vi "S2C_VLFT10_Proc_BoardPresent.vi"(8 "Error In":errorcluster, 11 "HandSwitch":T1 items=["Mono1 Cut", "Mono1 Coag", "Mono2 Cut", "Mono2 Coag", "Mono2 ValleyLab", "Bipolar", "LXF Bipolar", "Ligasure", "LXF Ligasure"]) -> (0 "Error Out":errorcluster, 3 "Present?":bool)   [LabVIEW 2015]
uses:
  Typedefs/S2C_VLFT10_Type_HandSwitch.ctl
  PCIe7841/VIs/Typedefs/S2C_PCIe7841_Type_PathRelayRd.ctl
  PCIe7841/VIs/Typedefs/S2C_PCIe7841_Type_RemRd.ctl
  PCIe7841/VIs/Typedefs/S2C_PCIe7841_Type_HandSwitchRd.ctl
  PCIe7841/VIs/Typedefs/S2C_PCIe7841_Type_SmokeEvacRd.ctl
  PCIe7841/VIs/PolyDriver/S2C_PCIe7841_Poly_RelayPathRead.vi
  PCIe7841/VIs/PolyDriver/S2C_PCIe7841_Poly_RemRead.vi
  PCIe7841/VIs/PolyDriver/S2C_PCIe7841_Poly_HandSwitchRead.vi
  PCIe7841/VIs/PolyDriver/S2C_PCIe7841_Poly_SmokeEvacRead.vi
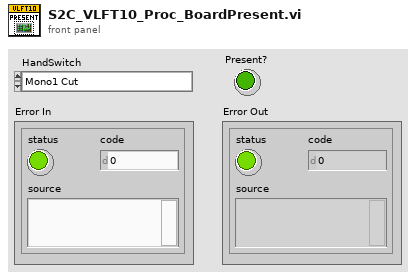
[diagram p1: front panel]
types:
  T1 = typedef "S2C_VLFT10_Type_HandSwitch.ctl" = u16
  T2 = typedef "S2C_PCIe7841_Type_HandSwitchRd.ctl" = string
  T3 = typedef "S2C_PCIe7841_Type_RemRd.ctl" = string
  T4 = typedef "S2C_PCIe7841_Type_PathRelayRd.ctl" = string
  T5 = typedef "S2C_PCIe7841_Type_SmokeEvacRd.ctl" = string
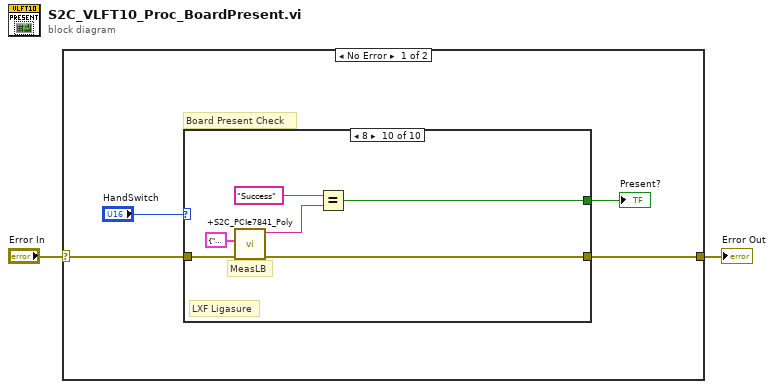
[diagram p0: block diagram]
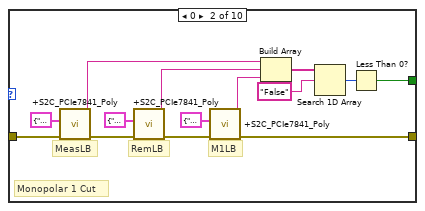
[diagram p3: hidden frame]
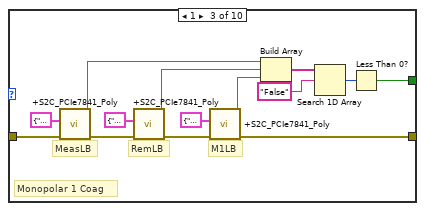
[diagram p4: hidden frame]
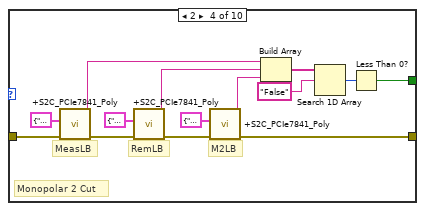
[diagram p5: hidden frame]
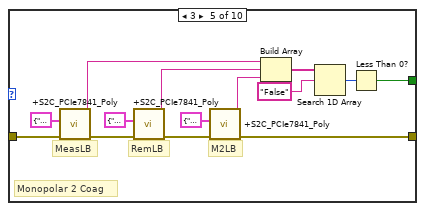
[diagram p6: hidden frame]
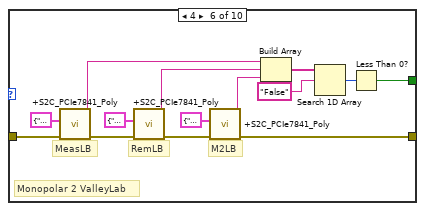
[diagram p7: hidden frame]
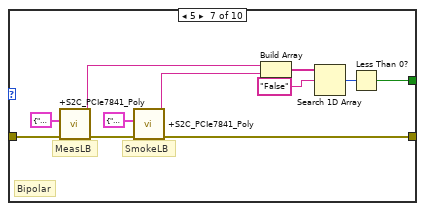
[diagram p8: hidden frame]
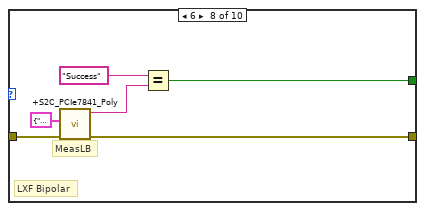
[diagram p9: hidden frame]
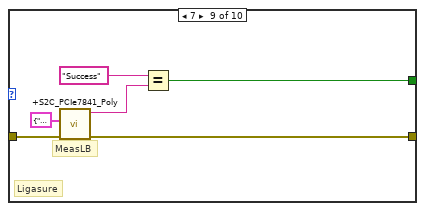
[diagram p10: hidden frame]
diagram:
  n1 = case shown="No Error" "Error In" {
    selector: "Error In" -> [w5 w107]
    tunnel: [w3 w107] -> w2
    frame No Error {
      # "Board Present Check"
      n2 = case shown="8" "HandSwitch" {
        tunnel: w5 -> [w7 w18 w32 w46 w60 w74 w87 w93 w99 w105]
        tunnel: [w7 w9 w23 w37 w51 w65 w79 w89 w95 w101] -> w3
        tunnel: [_ w8 w22 w36 w50 w64 w80 w92 w98 w104] -> w4
        frame 99, Default {
        }
        frame 0 {
          # "Monopolar 1 Cut"
          # "M1LB"
          # "RemLB"
          # "MeasLB"
          n3 = call-poly "+S2C_PCIe7841_Poly.vi"("Error In"=w18, "RelayPath"=cluster{"RelayPath":T4} {"RelayPath"="143"}) -> ("Error Out"=w17:errorcluster, "Response"=w15:string)  [unwired: 8 in]
          n4 = call-poly "+S2C_PCIe7841_Poly.vi"("Error In"=w17, "REM"=cluster{"REM":T3} {"REM"="123"}) -> ("Error Out"=w16:errorcluster, "Response"=w14:string)  [unwired: 8 in]
          n5 = call-poly "+S2C_PCIe7841_Poly.vi"("Error In"=w16, "HandSwitch"=cluster{"HandSwitch":T2} {"HandSwitch"="127"}) -> ("Error Out"=w9:errorcluster, "Response"=w13:string)  [unwired: 8 in]
          n6 = Build Array(w15, w14, w13) -> (w12:string[])
          n7 = Search 1D Array(1D array=w12, element="False") -> (index of element=w10:i32)  [unwired: 1 in]
          n8 = Less Than 0?(x=w10) -> (x < 0?=w8:bool)
        }
        frame 1 {
          # "Monopolar 1 Coag"
          # "M1LB"
          # "RemLB"
          # "MeasLB"
          n9 = call-poly "+S2C_PCIe7841_Poly.vi"("Error In"=w32, "RelayPath"=cluster{"RelayPath":T4} {"RelayPath"="143"}) -> ("Error Out"=w31:errorcluster, "Response"=w29:string)  [unwired: 8 in]
          n10 = call-poly "+S2C_PCIe7841_Poly.vi"("Error In"=w31, "REM"=cluster{"REM":T3} {"REM"="123"}) -> ("Error Out"=w30:errorcluster, "Response"=w28:string)  [unwired: 8 in]
          n11 = call-poly "+S2C_PCIe7841_Poly.vi"("Error In"=w30, "HandSwitch"=cluster{"HandSwitch":T2} {"HandSwitch"="127"}) -> ("Error Out"=w23:errorcluster, "Response"=w27:string)  [unwired: 8 in]
          n12 = Build Array(w29, w28, w27) -> (w26:string[])
          n13 = Search 1D Array(1D array=w26, element="False") -> (index of element=w24:i32)  [unwired: 1 in]
          n14 = Less Than 0?(x=w24) -> (x < 0?=w22:bool)
        }
        frame 2 {
          # "Monopolar 2 Cut"
          # "M2LB"
          # "RemLB"
          # "MeasLB"
          n15 = call-poly "+S2C_PCIe7841_Poly.vi"("Error In"=w46, "RelayPath"=cluster{"RelayPath":T4} {"RelayPath"="143"}) -> ("Error Out"=w45:errorcluster, "Response"=w43:string)  [unwired: 8 in]
          n16 = call-poly "+S2C_PCIe7841_Poly.vi"("Error In"=w45, "REM"=cluster{"REM":T3} {"REM"="123"}) -> ("Error Out"=w44:errorcluster, "Response"=w42:string)  [unwired: 8 in]
          n17 = call-poly "+S2C_PCIe7841_Poly.vi"("Error In"=w44, "HandSwitch"=cluster{"HandSwitch":T2} {"HandSwitch"="133"}) -> ("Error Out"=w37:errorcluster, "Response"=w41:string)  [unwired: 8 in]
          n18 = Build Array(w43, w42, w41) -> (w40:string[])
          n19 = Search 1D Array(1D array=w40, element="False") -> (index of element=w38:i32)  [unwired: 1 in]
          n20 = Less Than 0?(x=w38) -> (x < 0?=w36:bool)
        }
        frame 3 {
          # "Monopolar 2 Coag"
          # "M2LB"
          # "RemLB"
          # "MeasLB"
          n21 = call-poly "+S2C_PCIe7841_Poly.vi"("Error In"=w60, "RelayPath"=cluster{"RelayPath":T4} {"RelayPath"="143"}) -> ("Error Out"=w59:errorcluster, "Response"=w57:string)  [unwired: 8 in]
          n22 = call-poly "+S2C_PCIe7841_Poly.vi"("Error In"=w59, "REM"=cluster{"REM":T3} {"REM"="123"}) -> ("Error Out"=w58:errorcluster, "Response"=w56:string)  [unwired: 8 in]
          n23 = call-poly "+S2C_PCIe7841_Poly.vi"("Error In"=w58, "HandSwitch"=cluster{"HandSwitch":T2} {"HandSwitch"="133"}) -> ("Error Out"=w51:errorcluster, "Response"=w55:string)  [unwired: 8 in]
          n24 = Build Array(w57, w56, w55) -> (w54:string[])
          n25 = Search 1D Array(1D array=w54, element="False") -> (index of element=w52:i32)  [unwired: 1 in]
          n26 = Less Than 0?(x=w52) -> (x < 0?=w50:bool)
        }
        frame 4 {
          # "Monopolar 2 ValleyLab"
          # "M2LB"
          # "RemLB"
          # "MeasLB"
          n27 = call-poly "+S2C_PCIe7841_Poly.vi"("Error In"=w74, "RelayPath"=cluster{"RelayPath":T4} {"RelayPath"="143"}) -> ("Error Out"=w73:errorcluster, "Response"=w71:string)  [unwired: 8 in]
          n28 = call-poly "+S2C_PCIe7841_Poly.vi"("Error In"=w73, "REM"=cluster{"REM":T3} {"REM"="123"}) -> ("Error Out"=w72:errorcluster, "Response"=w70:string)  [unwired: 8 in]
          n29 = call-poly "+S2C_PCIe7841_Poly.vi"("Error In"=w72, "HandSwitch"=cluster{"HandSwitch":T2} {"HandSwitch"="133"}) -> ("Error Out"=w65:errorcluster, "Response"=w69:string)  [unwired: 8 in]
          n30 = Build Array(w71, w70, w69) -> (w68:string[])
          n31 = Search 1D Array(1D array=w68, element="False") -> (index of element=w66:i32)  [unwired: 1 in]
          n32 = Less Than 0?(x=w66) -> (x < 0?=w64:bool)
        }
        frame 5 {
          # "Bipolar"
          # "SmokeLB"
          # "MeasLB"
          n33 = call-poly "+S2C_PCIe7841_Poly.vi"("Error In"=w87, "RelayPath"=cluster{"RelayPath":T4} {"RelayPath"="143"}) -> ("Error Out"=w86:errorcluster, "Response"=w85:string)  [unwired: 8 in]
          n34 = call-poly "+S2C_PCIe7841_Poly.vi"("Error In"=w86, "SmokeEvac"=cluster{"SmokeEvac":T5} {"SmokeEvac"="137"}) -> ("Error Out"=w79:errorcluster, "Response"=w84:string)  [unwired: 8 in]
          n35 = Build Array(w85, w84) -> (w83:string[])
          n36 = Search 1D Array(1D array=w83, element="False") -> (index of element=w81:i32)  [unwired: 1 in]
          n37 = Less Than 0?(x=w81) -> (x < 0?=w80:bool)
        }
        frame 6 {
          # "LXF Bipolar"
          # "MeasLB"
          n38 = call-poly "+S2C_PCIe7841_Poly.vi"("Error In"=w93, "RelayPath"=cluster{"RelayPath":T4} {"RelayPath"="143"}) -> ("Error Out"=w89:errorcluster, "Response"=w91:string)  [unwired: 8 in]
          n39 = Equal?(x="Success", y=w91) -> (x = y?=w92:bool)
        }
        frame 7 {
          # "Ligasure"
          # "MeasLB"
          n40 = call-poly "+S2C_PCIe7841_Poly.vi"("Error In"=w99, "RelayPath"=cluster{"RelayPath":T4} {"RelayPath"="143"}) -> ("Error Out"=w95:errorcluster, "Response"=w97:string)  [unwired: 8 in]
          n41 = Equal?(x="Success", y=w97) -> (x = y?=w98:bool)
        }
        frame 8 {
          # "LXF Ligasure"
          # "MeasLB"
          n42 = call-poly "+S2C_PCIe7841_Poly.vi"("Error In"=w105, "RelayPath"=cluster{"RelayPath":T4} {"RelayPath"="143"}) -> ("Error Out"=w101:errorcluster, "Response"=w103:string)  [unwired: 8 in]
          n43 = Equal?(x="Success", y=w103) -> (x = y?=w104:bool)
        }
      }
      "Present?" <- w4
    }
    frame Error {
    }
  }
  "Error Out" <- w2
